vi "Syslog Collector - VS CD debug.vi"() -> (11 "Log File":path=path "c:/syslog.txt")   [LabVIEW 2016]
doc: "This VI illustrates using the Syslog reference design library to implement a Syslog collector application."
uses:
  <vilib>/NI/syslog/_subVIs/TypeDefs/syslog_message_cluster.ctl
  <vilib>/NI/syslog/_subVIs/TypeDefs/syslog_facility_codes.ctl
  <vilib>/NI/syslog/_subVIs/TypeDefs/syslog_severity_codes.ctl
panel:
  out "value":cluster{"Outputs":dbl[], "Inputs":dbl[]}
  out "error out":errorcluster
  out "Collector IP Address":string
  in  "Tab Control":enum32{"Syslog Collector", "Log File"}(tab)
  out "Messages Received":string
  out "Syslog Message":T1={"Facility Code"=enum."user", "Severity Code"=enum."emergency", "Time Stamp"=timestamp(0 s since 1904-01-01), "Hostname"="", "Message Tag"="", "Message Content"=""} {"Time Stamp" format="%<%I:%M:%S %p\n%m/%d>T"}
  out "Content":string
  in  "stop":bool
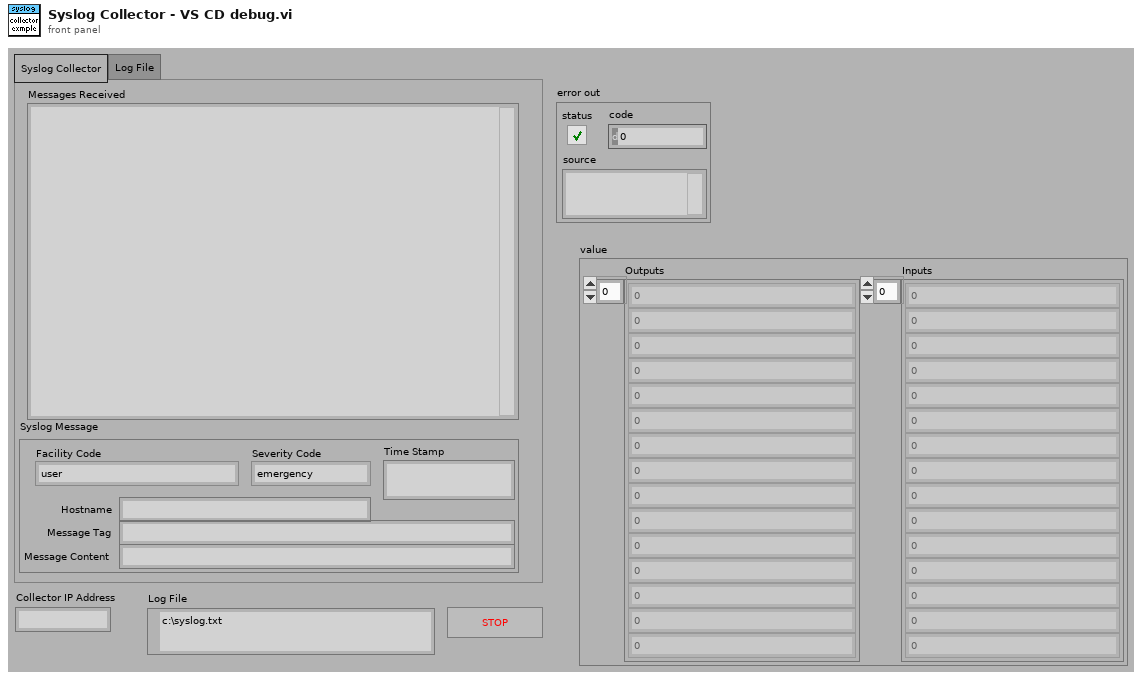
[diagram p1: front panel]
types:
  T1 = typedef "syslog_message_cluster.ctl" = cluster{"Facility Code":T2, "Severity Code":T3, "Time Stamp":timestamp, "Hostname":string, "Message Tag":string, "Message Content":string}
  T2 = typedef "syslog_facility_codes.ctl" = enum16{"kernel", "user", "mail", "system daemons", "security/authorization", "syslogd", "line printer", "network news", "uucp", "clock daemon", "security/authorization (alternate)", "FTP daemon", "NTP subsystem", "log audit", "log alert", "clock daemon (alternate)", "local use 0", "local use 1", "local use 2", "local use 3", "local use 4", "local use 5", "local use 6", "local use 7"}
  T3 = typedef "syslog_severity_codes.ctl" = enum16{"emergency", "alert", "critical", "error", "warning", "notice", "info", "debug"}
  T4 = enum16{"open", "replace", "create", "open or create", "replace or create", "replace or create with confirmation"}
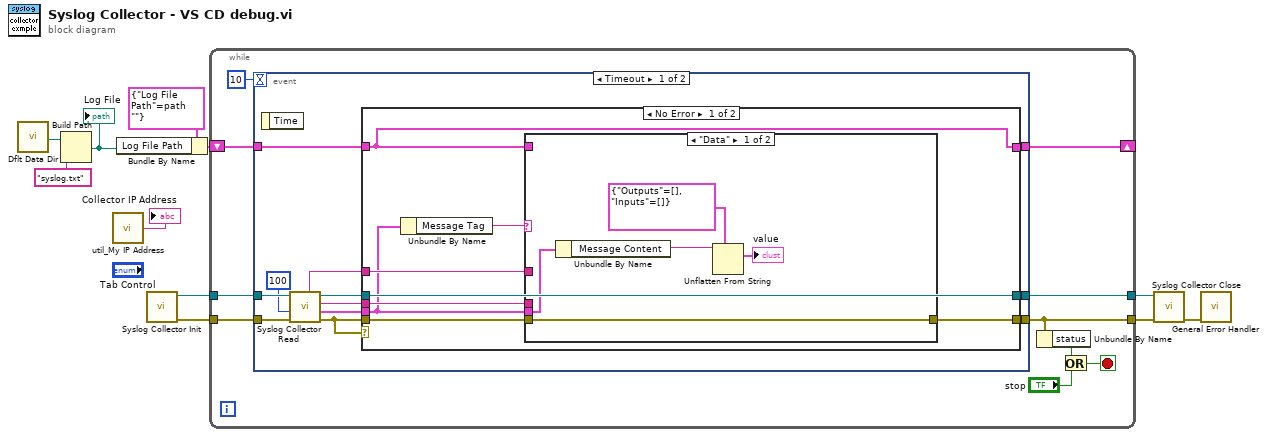
[diagram p0: block diagram]
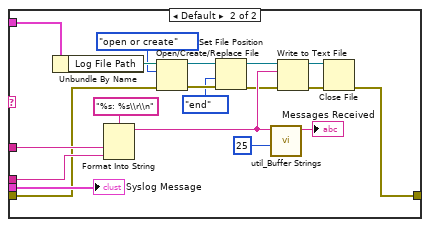
[diagram p2: hidden frame]
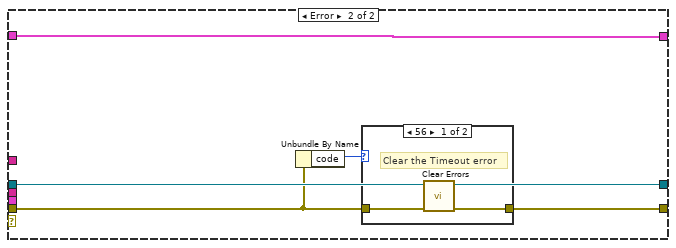
[diagram p3: hidden frame]
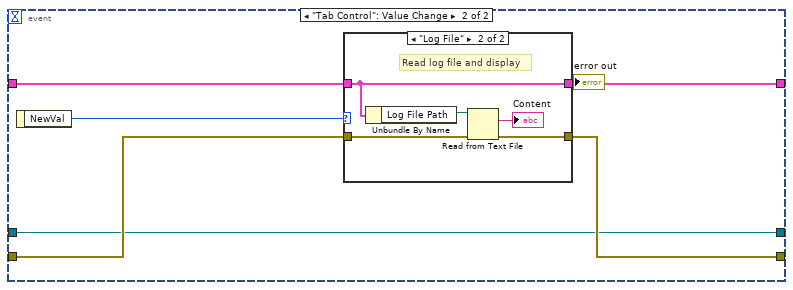
[diagram p5: hidden frame]
diagram:
  n1 = call <vilib>:"Dflt Data Dir.vi"() -> ("App:Default Data Directory"=w3:path)
  n2 = Build Path(base path=w3, name or relative path="syslog.txt") -> (appended path=w1:path)
  "Log File" <- w1
  n3 = call <vilib>:"util_My IP Address.vi"() -> ("IP Address"=→"Collector IP Address":string)  [unwired: 1 in]
  n4 = Bundle By Name(cluster=cluster{"Log File Path":path} {"Log File Path"=path ""} ("Cluster"), "Log File Path"=w1) -> (w9:cluster{"Log File Path":path})
  n5 = call <vilib>:"Syslog Collector Init.vi"() -> ("error out"=w10:errorcluster, "Syslog Collector Ref"=w11:refnum<k16>)  [unwired: 10 in]
  n6 = while {
    tunnel: w11 -> [w20]
    tunnel: w10 -> [w21]
    tunnel: [w19] -> w7
    shift-right: [w18] -> _
    shift-left: w9 -> [w16]
    tunnel: [w15] -> w5
    stop <- w12 stop-if-true
    n7 = event shown="[0] Timeout" {
      selector: _ -> [_ _]
      dyn-events: _ -> [_ _]
      timeout: 10 -> [_ _]
      tunnel: w21 -> [w33 w77]
      tunnel: w20 -> [w32 w74]
      tunnel: [w30 w74] -> w19
      tunnel: [w29 w75] -> w18
      tunnel: [w27 w76] -> w15
      tunnel: w16 -> [w23 w78]
      event Timeout {
        n8 = event-data() -> ()  [unwired: 1 in, 1 out]
        n9 = call <vilib>:"Syslog Collector Read.vi"("error in"=w33, "timeout ms (1000)"=100, "Syslog Collector Ref"=w32) -> ("error out"=w28:errorcluster, "syslog message cluster"=w24:T1, "syslog message"=w31:string, "Syslog Collector Ref"=w25:refnum<k16>, "syslog client address"=w26:string)  [unwired: 4 in]
        n10 = case shown="No Error" w28 {
          tunnel: w31 -> [w38 _]
          tunnel: [w41 w70] -> w30
          tunnel: w25 -> [w41 w70]
          tunnel: w23 -> [w40 w69]
          tunnel: [w40 w69] -> w29
          tunnel: [w36 w68] -> w27
          tunnel: w28 -> [w37 w67]
          tunnel: w26 -> [w39 _]
          tunnel: w24 -> [w35 _]
          frame No Error {
            n11 = Unbundle By Name(w35) -> ("Message Tag"=w34:string)
            n12 = case shown="\"Data\"" w34 {
              tunnel: w40 -> [_ w64]
              tunnel: w35 -> [w46 w61]
              tunnel: w39 -> [_ w58]
              tunnel: w38 -> [_ w57]
              tunnel: w37 -> [w45 w48]
              tunnel: [w45 w47] -> w36
              frame "Data" {
                n13 = Unbundle By Name(w46) -> ("Message Content"=w44:string)
                n14 = Unflatten From String(type=cluster{"Outputs":dbl[], "Inputs":dbl[]} {"Outputs"=[], "Inputs"=[]} ("Cluster"), binary string=w44) -> (value=→"value":cluster{"Outputs":dbl[], "Inputs":dbl[]})  [unwired: 3 in, 2 out]
              }
              frame Default {
                n15 = Unbundle By Name(w64) -> ("Log File Path"=w65:path)
                n16 = Format Into String(format string="%s: %s\\r\\n" ("string"), w58, w57) -> (resulting string=w60:string)  [unwired: 2 in, 1 out]
                n17 = Open/Create/Replace File(file path (use dialog)=w65, error in=w48, operation (0:open)=T4."open or create") -> (refnum out=w53:refnum<file>, error out=w54:errorcluster)  [unwired: 3 in, 1 out]
                n18 = Set File Position(refnum=w53, from (0:start)=enum16{"start", "end", "current"}."end", error in=w54) -> (refnum out=w52:refnum<file>, error out=w55:errorcluster)  [unwired: 1 in]
                n19 = call <vilib>:"util_Buffer Strings.vi"("Number of Strings to Buffer"=u8 25, "New String"=w60) -> ("Buffered String Series"=→"Messages Received":string)  [unwired: 9 in]
                n20 = Write to Text File(file (use dialog)=w52, text=w60, error in=w55) -> (refnum out=w50:refnum<file>, error out=w49:errorcluster)  [unwired: 1 in, 1 out]
                n21 = Close File(refnum=w50, error in=w49) -> (error out=w47:errorcluster)  [unwired: 1 out]
                "Syslog Message" <- w61
              }
            }
          }
          frame Error {
            n22 = Unbundle By Name(w67) -> ("code"=w66:i32)
            n23 = case shown="56" w66 {
              tunnel: w67 -> [w72 w73]
              tunnel: [w71 w73] -> w68
              frame 56 {
                # "Clear the Timeout error"
                n24 = call <vilib>:"Clear Errors.vi"("error in (no error)"=w72) -> ("error out"=w71:errorcluster)  [unwired: 5 in, 1 out]
              }
              frame Default {
              }
            }
          }
        }
      }
      event "Tab Control": Value Change {
        n25 = event-data() -> ("NewVal"=w79:enum32{"Syslog Collector", "Log File"})  [unwired: 1 in]
        n26 = case shown="\"Log File\"" w79 {
          tunnel: w78 -> [w80 w82]
          tunnel: w77 -> [w81 w84]
          tunnel: [w81 w83] -> w76
          tunnel: [w80 w82] -> w75
          frame "Syslog Collector", Default {
          }
          frame "Log File" {
            # "Read log file and display"
            n27 = Unbundle By Name(w82) -> ("Log File Path"=w86:path)
            n28 = Read from Text File(file (use dialog)=w86, error in=w84) -> (text=→"Content":string, error out=w83:errorcluster)  [unwired: 2 in, 2 out]
          }
        }
      }
    }
    n29 = Unbundle By Name(w15) -> ("status"=w14:bool)
    n30 = Or(x=w14, y="stop") -> (x .or. y?=w12:bool)
  }
  n31 = call <vilib>:"Syslog Collector Close.vi"("error in"=w5, "Syslog Collector Ref"=w7) -> ("error out"=w4:errorcluster)  [unwired: 9 in]
  n32 = call <vilib>:"General Error Handler.vi"("error in (no error)"=w4) -> ()  [unwired: 10 in, 5 out]
